vi "acquireMusic.vi"() -> ()   [LabVIEW 2018]
panel:
  in  "?":bool
  out "Collected Signals":dynamicdata(graph)
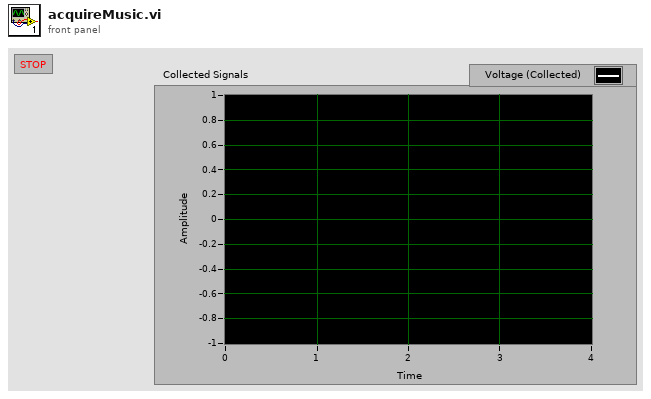
[diagram p1: front panel]
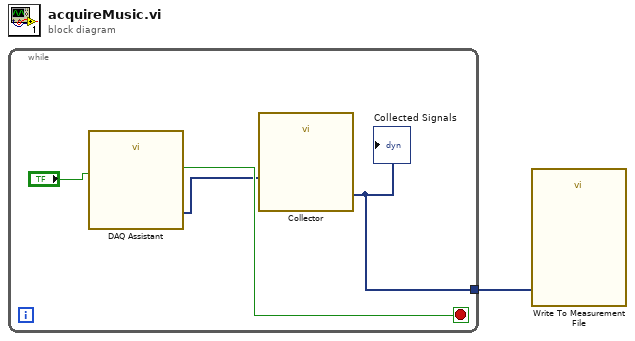
[diagram p0: block diagram]
diagram:
  n1 = while {
    tunnel: [w4] -> w1
    stop <- w3 stop-if-true
    n2 = call "DAQ Assistant"("stop (F)"="?") -> ("data"=w2:dynamicdata, "stopped"=w3:bool)  [unwired: 15 in, 2 out]
    n3 = call "Collector"("Signals"=w2) -> ("Collected Signals"=w4:dynamicdata)  [unwired: 9 in, 1 out]
    "Collected Signals" <- w4
  }
  n4 = call "Write To Measurement File"("Signals"=w1) -> ()  [unwired: 16 in, 3 out]
